vi "Validate Report Reference.vi"(0 "Report Ref In":T1, 1 "error in (no error)":errorcluster) -> (2 "Report Ref Out":T1, 3 "Valid":bool, 4 "error out":errorcluster)   [LabVIEW 2013, in "XCel Report Engine.lvlib"]
doc: "Validates a Report Ref before it is used by an XCelReportEngine operation.\n\nThis private helper verifies that the .NET API reference is valid and that the report session identifier represents an open session. If validation fails, it returns an error and prevents the requested operation from executing.\n\nIt is intended for internal use by the report engine library and should not be called directly by application code."
uses:
  XCel Report Engine.lvlib
  C:/Users/m.santucci/Documents/ChatGPT/LV_REPORT_ENGINE/LV/DotNet/XCelReportEngine.dll
  LV/DotNet/XCelReportEngine.dll
  Controls/Report Ref.ctl
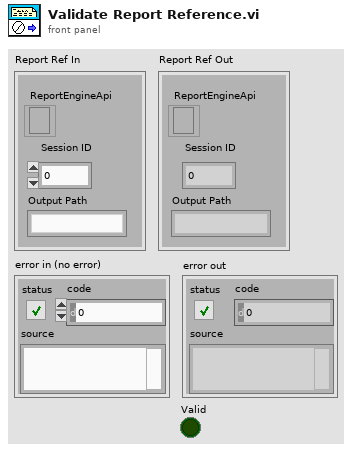
[diagram p1: front panel]
types:
  T1 = typedef "XCel Report Engine.lvlib/Report Ref.ctl" = cluster{"Session ID":i32, "Output Path":string, "ReportEngineApi":refnum<k24>}
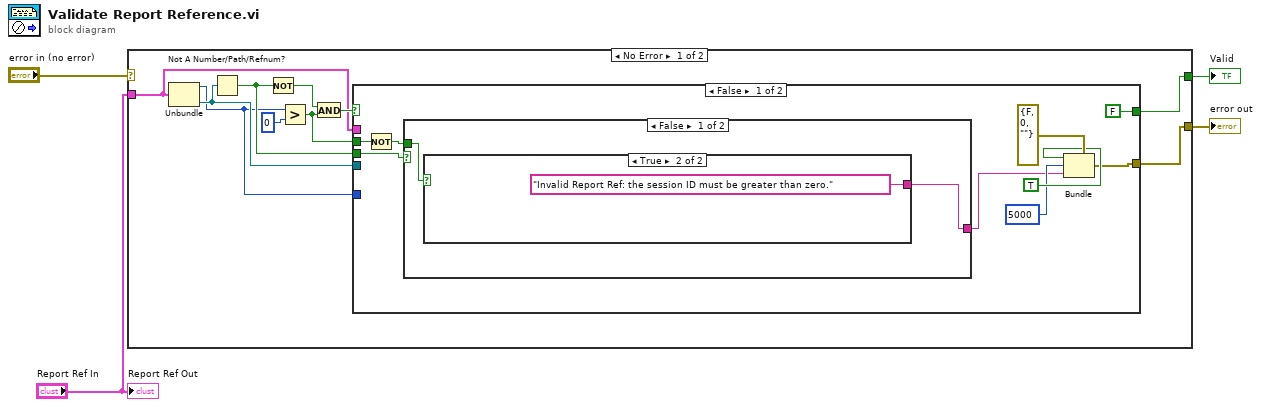
[diagram p0: block diagram]
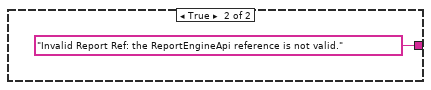
[diagram p3: hidden frame]
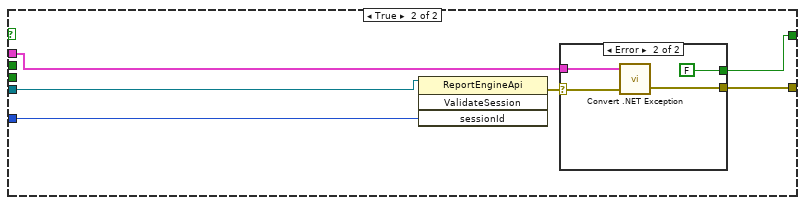
[diagram p4: hidden frame]
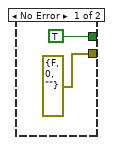
[diagram p5: hidden frame]
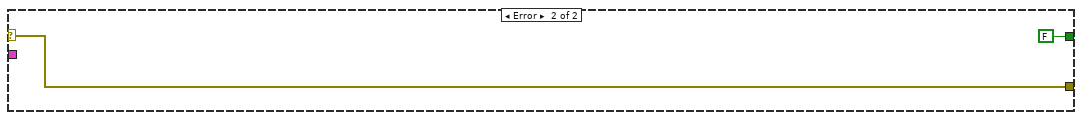
[diagram p6: hidden frame]
diagram:
  n1 = case shown="No Error" "error in (no error)" {
    selector: "error in (no error)" -> [_ w41]
    tunnel: "Report Ref In" -> [w11 _]
    tunnel: [w13 FALSE ("Valid")] -> w3
    tunnel: [w12 w41] -> w2
    frame No Error {
      n2 = Unbundle(w11) -> ("Session ID"=w5:i32, "ReportEngineApi"=w10:refnum<k24>)  [unwired: 1 out]
      n3 = Not A Number/Path/Refnum?(number/path/refnum=w10) -> (NaN/Path/Refnum?=w9:bool)
      n4 = Not(x=w9) -> (.not. x?=w8:bool)
      n5 = Greater?(x=w5, y=0 ("x")) -> (0:w7:bool)
      n6 = And(x=w8, y=w7) -> (x .and. y?=w14:bool)
      n7 = case shown="False" w14 {
        tunnel: w5 -> [_ w33]
        tunnel: [FALSE ("Valid") w31] -> w13
        tunnel: [w15 w30] -> w12
        tunnel: w7 -> [w22 _]
        tunnel: w11 -> [_ w29]
        tunnel: w10 -> [_ w28]
        tunnel: w9 -> [w21 _]
        frame False {
          n8 = Not(x=w22) -> (.not. x?=w16:bool)
          n9 = case shown="False" w21 {
            tunnel: [w24 "Invalid Report Ref: the ReportEngineApi reference is not valid."] -> w17
            tunnel: w16 -> [w25 _]
            frame False {
              n10 = case shown="True" w25 {
                tunnel: [_ "Invalid Report Ref: the session ID must be greater than zero."] -> w24
                frame False {
                }
                frame True {
                }
              }
            }
            frame True {
            }
          }
          n11 = Bundle(cluster=errorcluster {"status"=FALSE, "code"=0, "source"=""} ("error IO"), "status"=TRUE, "code"=5000, "source"=w17) -> (w15:errorcluster)
        }
        frame True {
          n12 = invoke class="ReportEngineApi" method="ValidateSession"(reference=w28, "sessionId"=w33) -> (error out=w32:errorcluster)  [unwired: 2 in, 3 out]
          n13 = case shown="Error" w32 {
            selector: w32 -> [_ w38]
            tunnel: [TRUE ("Valid") FALSE ("Valid")] -> w31
            tunnel: [errorcluster {"status"=FALSE, "code"=0, "source"=""} ("error IO") w37] -> w30
            tunnel: w29 -> [_ w36]
            frame No Error {
            }
            frame Error {
              n14 = call "Convert .NET Exception.vi"("error in (no error)"=w38, "Report Ref In"=w36) -> ("error out"=w37:errorcluster)  [unwired: 1 in, 1 out]
            }
          }
        }
      }
    }
    frame Error {
    }
  }
  "Valid" <- w3
  "error out" <- w2
  "Report Ref Out" <- "Report Ref In"
